vi "onBoard LED.vi"(8 "Error In":errorcluster, 11 "LED[3:0]":u8 format="%.0b") -> (0 "Error Out":errorcluster)   [LabVIEW 2019]
uses:
  FPGA/FPGA varible.vi
  <vilib>/Utility/error.llb/Error Cluster From Error Code.vi
  <vilib>/rvi/errors/niLvFpgaAdjustHostInterfaceError.vi
  <vilib>/rvi/interface/nirviReadWriteControl/nirviReadWriteControl.xnode
  NiFpgaLv.dll
  <vilib>/rvi/interface/Simulation/niFpgaSimulationCallBeginRW.vi
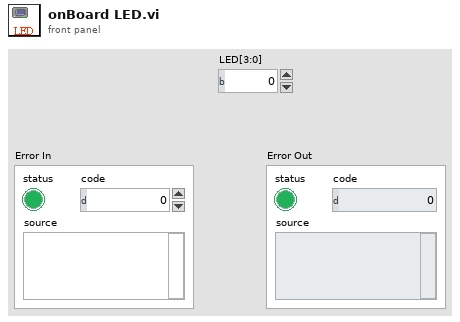
[diagram p1: front panel]
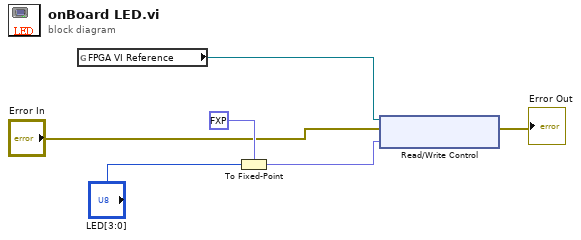
[diagram p0: block diagram]
diagram:
  n1 = global read "FPGA varible.vi" "FPGA VI Reference"() -> (w6:refnum<k20>)
  n2 = To Fixed-Point(fixed-point type=fxp<+,4,4> 0.0, number="LED[3:0]") -> (fixed-point=w4:fxp<+,4,4>)
  n3 = xnode "Read/Write Control"("FPGA VI Reference In"=w6, "error in"="Error In", "OnBoard.LED[3:0]"=w4) -> ("error out"=→"Error Out":errorcluster)  [unwired: 1 out]
